vi "test json performance.vi"(8 "error in (no error)":errorcluster) -> (0 "error out":errorcluster, 1 "ms Avg Dump":dbl, 2 "ms Avg Load":dbl, 3 "Passed?":bool)   [LabVIEW 2019, in "labview_json_tests.lvlib"]
uses:
  labview_json_tests.lvlib
  lib/labview_json.lvlib
panel:
  out "Variant out":variant
  out "JSON out":string
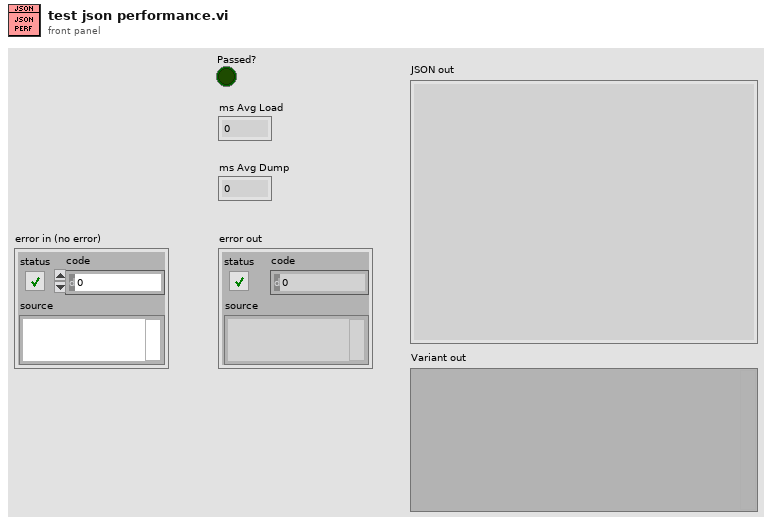
[diagram p1: front panel]
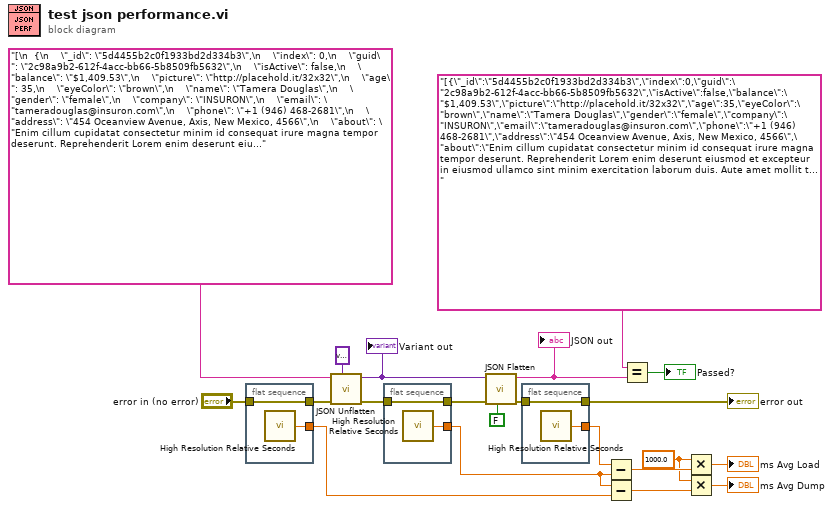
[diagram p0: block diagram]
diagram:
  w8 = 1000.0 ("x")
  n1 = flat-sequence {
    tunnel: [w23] -> w18
    tunnel: "error in (no error)" -> [w23]
    tunnel: [w22] -> w13
    frame #0 {
      n2 = call <vilib>:"High Resolution Relative Seconds.vi"() -> ("relative seconds"=w22:dbl)
    }
  }
  n3 = call "JSON Unflatten.vi"("Variant Type"=variant, "error in (no error)"=w18, "JSON in"="[\n  {\n    \"_id\": \"5d4455b2c0f1933bd2d334b3\",\n    \"index\": 0,\n    \"guid\": \"2c98a9b2-612f-4acc-bb66-5b8509fb5632\",\n    \"isActive\": false,\n    \"balance\": \"$1,409.53\",\n    \"picture\": \"http://placehold.it/32x32\",\n    \"age\": 35,\n    \"eyeColor\": \"brown\",\n    \"name\": \"Tamera Douglas\",\n    \"gender\": \"female\",\n    \"company\": \"INSURON\",\n    \"email\": \"tameradouglas@insuron.com\",\n    \"phone\": \"+1 (946) 468-2681\",\n    \"address\": \"454 Oceanview Avenue, Axis, New Mexico, 4566\",\n    \"about\": \"Enim cillum cupidatat consectetur minim id consequat irure magna tempor deserunt. Reprehenderit Lorem enim deserunt eiusmod et excepteur in eiusmod ullamco sint minim exercitation laborum duis. Aute amet mollit tempor adipisicing. Eiusmod tempor qui proident amet sint eiusmod laborum nisi consectetur. Excepteur occaecat et consequat pariatur pariatur sit deserunt proident commodo enim sit do. Duis fugiat irure esse ipsum non nulla ut aliquip esse nisi. Mollit commodo sit elit amet duis nisi sint.\",\n    \"registered\": \"2019-04-15T12:36:48 +06:00\",\n    \"latitude\": 7.38495,\n    \"longitude\": -44.890348,\n    \"tags\": [\n      \"cillum\",\n      \"nisi\",\n      \"mollit\",\n      \"sunt\",\n      \"minim\",\n      \"non\",\n      \"ex\"\n    ],\n    \"friends\": [\n      {\n        \"id\": 0,\n        \"name\": \"Winnie Reid\"\n      },\n      {\n        \"id\": 1,\n        \"name\": \"Araceli Delacruz\"\n      },\n      {\n        \"id\": 2,\n        \"name\": \"Bolton Horne\"\n      }\n    ],\n    \"greeting\": \"Hello, Tamera Douglas! You have 1 unread messages.\",\n    \"favoriteFruit\": \"banana\"\n  },\n  {\n    \"_id\": \"5d4455b247ae2b298863909d\",\n    \"index\": 1,\n    \"guid\": \"00a03766-a5ca-45cc-8dfb-1ef19cade6a5\",\n    \"isActive\": true,\n    \"balance\": \"$2,933.39\",\n    \"picture\": \"http://placehold.it/32x32\",\n    \"age\": 30,\n    \"eyeColor\": \"blue\",\n    \"name\": \"Garner Hooper\",\n    \"gender\": \"male\",\n    \"company\": \"SENMEI\",\n    \"email\": \"garnerhooper@senmei.com\",\n    \"phone\": \"+1 (805) 444-2443\",\n    \"address\": \"334 Herkimer Place, Westphalia, West Virginia, 8777\",\n    \"about\": \"Tempor tempor commodo do cillum ex. Velit minim esse nulla incididunt cupidatat. Aliqua tempor magna pariatur incididunt nostrud id cupidatat aliquip elit est ullamco. Mollit magna ut deserunt nisi exercitation reprehenderit proident ipsum occaecat ut enim. Voluptate adipisicing culpa veniam duis amet.\",\n    \"registered\": \"2019-02-20T09:03:35 +07:00\",\n    \"latitude\": 3.634789,\n    \"longitude\": -71.711449,\n    \"tags\": [\n      \"laboris\",\n      \"sunt\",\n      \"elit\",\n      \"esse\",\n      \"aliqua\",\n      \"nulla\",\n      \"in\"\n    ],\n    \"friends\": [\n      {\n        \"id\": 0,\n        \"name\": \"Saundra Mullen\"\n      },\n      {\n        \"id\": 1,\n        \"name\": \"Macdonald Houston\"\n      },\n      {\n        \"id\": 2,\n        \"name\": \"Rivera Hyde\"\n      }\n    ],\n    \"greeting\": \"Hello, Garner Hooper! You have 1 unread messages.\",\n    \"favoriteFruit\": \"banana\"\n  },\n  {\n    \"_id\": \"5d4455b288b3a8bcda8c1081\",\n    \"index\": 2,\n    \"guid\": \"14e7d77e-1ed5-4b08-bdae-19e0328d29f8\",\n    \"isActive\": false,\n    \"balance\": \"$1,321.03\",\n    \"picture\": \"http://placehold.it/32x32\",\n    \"age\": 33,\n    \"eyeColor\": \"blue\",\n    \"name\": \"Neal Buckley\",\n    \"gender\": \"male\",\n    \"company\": \"TRIBALOG\",\n    \"email\": \"nealbuckley@tribalog.com\",\n    \"phone\": \"+1 (879) 521-3254\",\n    \"address\": \"378 Preston Court, Unionville, Northern Mariana Islands, 6583\",\n    \"about\": \"Elit enim consectetur ad non tempor ad tempor proident do. In consectetur fugiat commodo ex. Ut nulla voluptate aliquip esse. Officia esse proident minim enim cillum deserunt mollit. Anim do deserunt amet velit consequat anim ullamco enim Lorem esse culpa irure voluptate labore. Laboris officia officia aliqua elit elit non culpa cillum dolore amet quis.\",\n    \"registered\": \"2019-01-23T03:40:45 +07:00\",\n    \"latitude\": 8.381404,\n    \"longitude\": -96.636286,\n    \"tags\": [\n      \"velit\",\n      \"esse\",\n      \"id\",\n      \"ullamco\",\n      \"sunt\",\n      \"amet\",\n      \"ad\"\n    ],\n    \"friends\": [\n      {\n        \"id\": 0,\n        \"name\": \"Hall Booker\"\n      },\n      {\n        \"id\": 1,\n        \"name\": \"Lawson Stevenson\"\n      },\n      {\n        \"id\": 2,\n        \"name\": \"Maynard Gill\"\n      }\n    ],\n    \"greeting\": \"Hello, Neal Buckley! You have 9 unread messages.\",\n    \"favoriteFruit\": \"apple\"\n  },\n  {\n    \"_id\": \"5d4455b21a3db63bef3f777a\",\n    \"index\": 3,\n    \"guid\": \"d4ea16a6-f1ec-4bfe-9970-657798a14ac1\",\n    \"isActive\": false,\n    \"balance\": \"$2,499.94\",\n    \"picture\": \"http://placehold.it/32x32\",\n    \"age\": 37,\n    \"eyeColor\": \"green\",\n    \"name\": \"Marguerite Gay\",\n    \"gender\": \"female\",\n    \"company\": \"DADABASE\",\n    \"email\": \"margueritegay@dadabase.com\",\n    \"phone\": \"+1 (937) 434-3754\",\n    \"address\": \"256 Dooley Street, Sylvanite, Nevada, 1343\",\n    \"about\": \"Aute elit laborum cillum minim esse ex eu est. Cillum in esse irure ut do duis et eiusmod aliqua et adipisicing. Sunt adipisicing commodo dolor sit qui laborum commodo deserunt amet minim. Proident sint labore consequat commodo enim veniam veniam ea amet eu qui. Officia culpa dolor adipisicing laborum. Commodo elit sunt anim laboris laborum amet nulla.\",\n    \"registered\": \"2014-05-27T12:57:25 +06:00\",\n    \"latitude\": 64.083884,\n    \"longitude\": -30.078651,\n    \"tags\": [\n      \"minim\",\n      \"mollit\",\n      \"laboris\",\n      \"pariatur\",\n      \"qui\",\n      \"sit\",\n      \"do\"\n    ],\n    \"friends\": [\n      {\n        \"id\": 0,\n        \"name\": \"Duffy Steele\"\n      },\n      {\n        \"id\": 1,\n        \"name\": \"Preston Lamb\"\n      },\n      {\n        \"id\": 2,\n        \"name\": \"Velasquez Shaffer\"\n      }\n    ],\n    \"greeting\": \"Hello, Marguerite Gay! You have 5 unread messages.\",\n    \"favoriteFruit\": \"apple\"\n  },\n  {\n    \"_id\": \"5d4455b2664446faf7994a00\",\n    \"index\": 4,\n    \"guid\": \"75fe4cd8-2ec4-47e4-9a35-4a72f803cd01\",\n    \"isActive\": true,\n    \"balance\": \"$3,522.35\",\n    \"picture\": \"http://placehold.it/32x32\",\n    \"age\": 20,\n    \"eyeColor\": \"brown\",\n    \"name\": \"Graciela Orr\",\n    \"gender\": \"female\",\n    \"company\": \"ENTROFLEX\",\n    \"email\": \"gracielaorr@entroflex.com\",\n    \"phone\": \"+1 (855) 541-3462\",\n    \"address\": \"895 Sapphire Street, Ruckersville, Georgia, 6484\",\n    \"about\": \"Consectetur reprehenderit laboris minim anim aute aliquip Lorem ullamco non consequat. Tempor officia occaecat eu amet quis quis fugiat. Eu ad ex elit dolor. Do proident veniam aute irure consectetur laborum nulla qui Lorem ut culpa commodo. Quis commodo commodo sint sunt veniam. Magna commodo reprehenderit duis eu deserunt qui amet. Pariatur ut occaecat minim officia commodo voluptate esse in id anim.\",\n    \"registered\": \"2017-02-22T08:24:12 +07:00\",\n    \"latitude\": -84.018578,\n    \"longitude\": 66.386099,\n    \"tags\": [\n      \"excepteur\",\n      \"anim\",\n      \"commodo\",\n      \"amet\",\n      \"consequat\",\n      \"tempor\",\n      \"quis\"\n    ],\n    \"friends\": [\n      {\n        \"id\": 0,\n        \"name\": \"Ollie Cline\"\n      },\n      {\n        \"id\": 1,\n        \"name\": \"Corina Powers\"\n      },\n      {\n        \"id\": 2,\n        \"name\": \"Lynda Workman\"\n      }\n    ],\n    \"greeting\": \"Hello, Graciela Orr! You have 6 unread messages.\",\n    \"favoriteFruit\": \"apple\"\n  },\n  {\n    \"_id\": \"5d4455b2ca59b0a7fc9c71cd\",\n    \"index\": 5,\n    \"guid\": \"a5d705b7-9c22-4a73-968c-37b6847d31de\",\n    \"isActive\": true,\n    \"balance\": \"$2,719.98\",\n    \"picture\": \"http://placehold.it/32x32\",\n    \"age\": 30,\n    \"eyeColor\": \"blue\",\n    \"name\": \"Lynn Durham\",\n    \"gender\": \"male\",\n    \"company\": \"RODEOMAD\",\n    \"email\": \"lynndurham@rodeomad.com\",\n    \"phone\": \"+1 (896) 522-2325\",\n    \"address\": \"202 Erskine Loop, Silkworth, North Dakota, 8325\",\n    \"about\": \"Anim sunt irure ut sint. Ullamco consectetur non pariatur consectetur ullamco. Consequat cupidatat nisi eiusmod magna ut eiusmod. Ullamco cillum culpa voluptate fugiat laboris nulla Lorem ad irure ipsum mollit.\",\n    \"registered\": \"2017-06-19T08:42:14 +06:00\",\n    \"latitude\": -19.936145,\n    \"longitude\": 149.259571,\n    \"tags\": [\n      \"ea\",\n      \"proident\",\n      \"tempor\",\n      \"cillum\",\n      \"sit\",\n      \"veniam\",\n      \"velit\"\n    ],\n    \"friends\": [\n      {\n        \"id\": 0,\n        \"name\": \"Horne Kelley\"\n      },\n      {\n        \"id\": 1,\n        \"name\": \"Elvia Harper\"\n      },\n      {\n        \"id\": 2,\n        \"name\": \"Hooper Griffith\"\n      }\n    ],\n    \"greeting\": \"Hello, Lynn Durham! You have 2 unread messages.\",\n    \"favoriteFruit\": \"banana\"\n  },\n  {\n    \"_id\": \"5d4455b2293b6080ad5e354a\",\n    \"index\": 6,\n    \"guid\": \"64e7c98c-aecf-4ff2-aeff-e95c9629e4fa\",\n    \"isActive\": false,\n    \"balance\": \"$3,702.37\",\n    \"picture\": \"http://placehold.it/32x32\",\n    \"age\": 22,\n    \"eyeColor\": \"brown\",\n    \"name\": \"Bethany Salazar\",\n    \"gender\": \"female\",\n    \"company\": \"TRIPSCH\",\n    \"email\": \"bethanysalazar@tripsch.com\",\n    \"phone\": \"+1 (856) 524-3649\",\n    \"address\": \"754 Prospect Place, Crumpler, Palau, 1899\",\n    \"about\": \"Tempor non occaecat veniam non. Mollit exercitation magna eiusmod cillum. Consequat do irure deserunt velit. Consectetur aute deserunt esse anim nostrud do.\",\n    \"registered\": \"2014-09-10T09:21:42 +06:00\",\n    \"latitude\": -55.3388,\n    \"longitude\": -63.497523,\n    \"tags\": [\n      \"incididunt\",\n      \"cupidatat\",\n      \"voluptate\",\n      \"pariatur\",\n      \"dolore\",\n      \"tempor\",\n      \"laborum\"\n    ],\n    \"friends\": [\n      {\n        \"id\": 0,\n        \"name\": \"Weiss Hahn\"\n      },\n      {\n        \"id\": 1,\n        \"name\": \"Trudy Roy\"\n      },\n      {\n        \"id\": 2,\n        \"name\": \"Schultz Vazquez\"\n      }\n    ],\n    \"greeting\": \"Hello, Bethany Salazar! You have 4 unread messages.\",\n    \"favoriteFruit\": \"banana\"\n  }\n]" ("JSON")) -> ("error out"=w17:errorcluster, "Variant out"=w14:variant)  [unwired: 6 in, 1 out]
  "Variant out" <- w14
  n4 = flat-sequence {
    tunnel: [w25] -> w16
    tunnel: w17 -> [w25]
    tunnel: [w24] -> w11
    frame #0 {
      n5 = call <vilib>:"High Resolution Relative Seconds.vi"() -> ("relative seconds"=w24:dbl)
    }
  }
  n6 = call "JSON Flatten.vi"("Pretty Print? (F)"=FALSE, "error in (no error)"=w16, "Variant in"=w14) -> ("error out"=w15:errorcluster, "JSON out"=w20:string)  [unwired: 7 in]
  "JSON out" <- w20
  n7 = flat-sequence {
    tunnel: [w27] -> w2
    tunnel: w15 -> [w27]
    tunnel: [w26] -> w12
    frame #0 {
      n8 = call <vilib>:"High Resolution Relative Seconds.vi"() -> ("relative seconds"=w26:dbl)
    }
  }
  n9 = Subtract(x=w12, y=w11) -> (x-y=w10:dbl)
  n10 = Subtract(x=w11, y=w13) -> (x-y=w9:dbl)
  n11 = Equal?(x="[{\"_id\":\"5d4455b2c0f1933bd2d334b3\",\"index\":0,\"guid\":\"2c98a9b2-612f-4acc-bb66-5b8509fb5632\",\"isActive\":false,\"balance\":\"$1,409.53\",\"picture\":\"http://placehold.it/32x32\",\"age\":35,\"eyeColor\":\"brown\",\"name\":\"Tamera Douglas\",\"gender\":\"female\",\"company\":\"INSURON\",\"email\":\"tameradouglas@insuron.com\",\"phone\":\"+1 (946) 468-2681\",\"address\":\"454 Oceanview Avenue, Axis, New Mexico, 4566\",\"about\":\"Enim cillum cupidatat consectetur minim id consequat irure magna tempor deserunt. Reprehenderit Lorem enim deserunt eiusmod et excepteur in eiusmod ullamco sint minim exercitation laborum duis. Aute amet mollit tempor adipisicing. Eiusmod tempor qui proident amet sint eiusmod laborum nisi consectetur. Excepteur occaecat et consequat pariatur pariatur sit deserunt proident commodo enim sit do. Duis fugiat irure esse ipsum non nulla ut aliquip esse nisi. Mollit commodo sit elit amet duis nisi sint.\",\"registered\":\"2019-04-15T12:36:48 +06:00\",\"latitude\":7.38495,\"longitude\":-44.890348,\"tags\":[\"cillum\",\"nisi\",\"mollit\",\"sunt\",\"minim\",\"non\",\"ex\"],\"friends\":[{\"id\":0,\"name\":\"Winnie Reid\"},{\"id\":1,\"name\":\"Araceli Delacruz\"},{\"id\":2,\"name\":\"Bolton Horne\"}],\"greeting\":\"Hello, Tamera Douglas! You have 1 unread messages.\",\"favoriteFruit\":\"banana\"},{\"_id\":\"5d4455b247ae2b298863909d\",\"index\":1,\"guid\":\"00a03766-a5ca-45cc-8dfb-1ef19cade6a5\",\"isActive\":true,\"balance\":\"$2,933.39\",\"picture\":\"http://placehold.it/32x32\",\"age\":30,\"eyeColor\":\"blue\",\"name\":\"Garner Hooper\",\"gender\":\"male\",\"company\":\"SENMEI\",\"email\":\"garnerhooper@senmei.com\",\"phone\":\"+1 (805) 444-2443\",\"address\":\"334 Herkimer Place, Westphalia, West Virginia, 8777\",\"about\":\"Tempor tempor commodo do cillum ex. Velit minim esse nulla incididunt cupidatat. Aliqua tempor magna pariatur incididunt nostrud id cupidatat aliquip elit est ullamco. Mollit magna ut deserunt nisi exercitation reprehenderit proident ipsum occaecat ut enim. Voluptate adipisicing culpa veniam duis amet.\",\"registered\":\"2019-02-20T09:03:35 +07:00\",\"latitude\":3.634789,\"longitude\":-71.711449,\"tags\":[\"laboris\",\"sunt\",\"elit\",\"esse\",\"aliqua\",\"nulla\",\"in\"],\"friends\":[{\"id\":0,\"name\":\"Saundra Mullen\"},{\"id\":1,\"name\":\"Macdonald Houston\"},{\"id\":2,\"name\":\"Rivera Hyde\"}],\"greeting\":\"Hello, Garner Hooper! You have 1 unread messages.\",\"favoriteFruit\":\"banana\"},{\"_id\":\"5d4455b288b3a8bcda8c1081\",\"index\":2,\"guid\":\"14e7d77e-1ed5-4b08-bdae-19e0328d29f8\",\"isActive\":false,\"balance\":\"$1,321.03\",\"picture\":\"http://placehold.it/32x32\",\"age\":33,\"eyeColor\":\"blue\",\"name\":\"Neal Buckley\",\"gender\":\"male\",\"company\":\"TRIBALOG\",\"email\":\"nealbuckley@tribalog.com\",\"phone\":\"+1 (879) 521-3254\",\"address\":\"378 Preston Court, Unionville, Northern Mariana Islands, 6583\",\"about\":\"Elit enim consectetur ad non tempor ad tempor proident do. In consectetur fugiat commodo ex. Ut nulla voluptate aliquip esse. Officia esse proident minim enim cillum deserunt mollit. Anim do deserunt amet velit consequat anim ullamco enim Lorem esse culpa irure voluptate labore. Laboris officia officia aliqua elit elit non culpa cillum dolore amet quis.\",\"registered\":\"2019-01-23T03:40:45 +07:00\",\"latitude\":8.381404,\"longitude\":-96.636286,\"tags\":[\"velit\",\"esse\",\"id\",\"ullamco\",\"sunt\",\"amet\",\"ad\"],\"friends\":[{\"id\":0,\"name\":\"Hall Booker\"},{\"id\":1,\"name\":\"Lawson Stevenson\"},{\"id\":2,\"name\":\"Maynard Gill\"}],\"greeting\":\"Hello, Neal Buckley! You have 9 unread messages.\",\"favoriteFruit\":\"apple\"},{\"_id\":\"5d4455b21a3db63bef3f777a\",\"index\":3,\"guid\":\"d4ea16a6-f1ec-4bfe-9970-657798a14ac1\",\"isActive\":false,\"balance\":\"$2,499.94\",\"picture\":\"http://placehold.it/32x32\",\"age\":37,\"eyeColor\":\"green\",\"name\":\"Marguerite Gay\",\"gender\":\"female\",\"company\":\"DADABASE\",\"email\":\"margueritegay@dadabase.com\",\"phone\":\"+1 (937) 434-3754\",\"address\":\"256 Dooley Street, Sylvanite, Nevada, 1343\",\"about\":\"Aute elit laborum cillum minim esse ex eu est. Cillum in esse irure ut do duis et eiusmod aliqua et adipisicing. Sunt adipisicing commodo dolor sit qui laborum commodo deserunt amet minim. Proident sint labore consequat commodo enim veniam veniam ea amet eu qui. Officia culpa dolor adipisicing laborum. Commodo elit sunt anim laboris laborum amet nulla.\",\"registered\":\"2014-05-27T12:57:25 +06:00\",\"latitude\":64.083884,\"longitude\":-30.078651,\"tags\":[\"minim\",\"mollit\",\"laboris\",\"pariatur\",\"qui\",\"sit\",\"do\"],\"friends\":[{\"id\":0,\"name\":\"Duffy Steele\"},{\"id\":1,\"name\":\"Preston Lamb\"},{\"id\":2,\"name\":\"Velasquez Shaffer\"}],\"greeting\":\"Hello, Marguerite Gay! You have 5 unread messages.\",\"favoriteFruit\":\"apple\"},{\"_id\":\"5d4455b2664446faf7994a00\",\"index\":4,\"guid\":\"75fe4cd8-2ec4-47e4-9a35-4a72f803cd01\",\"isActive\":true,\"balance\":\"$3,522.35\",\"picture\":\"http://placehold.it/32x32\",\"age\":20,\"eyeColor\":\"brown\",\"name\":\"Graciela Orr\",\"gender\":\"female\",\"company\":\"ENTROFLEX\",\"email\":\"gracielaorr@entroflex.com\",\"phone\":\"+1 (855) 541-3462\",\"address\":\"895 Sapphire Street, Ruckersville, Georgia, 6484\",\"about\":\"Consectetur reprehenderit laboris minim anim aute aliquip Lorem ullamco non consequat. Tempor officia occaecat eu amet quis quis fugiat. Eu ad ex elit dolor. Do proident veniam aute irure consectetur laborum nulla qui Lorem ut culpa commodo. Quis commodo commodo sint sunt veniam. Magna commodo reprehenderit duis eu deserunt qui amet. Pariatur ut occaecat minim officia commodo voluptate esse in id anim.\",\"registered\":\"2017-02-22T08:24:12 +07:00\",\"latitude\":-84.018578,\"longitude\":66.386099,\"tags\":[\"excepteur\",\"anim\",\"commodo\",\"amet\",\"consequat\",\"tempor\",\"quis\"],\"friends\":[{\"id\":0,\"name\":\"Ollie Cline\"},{\"id\":1,\"name\":\"Corina Powers\"},{\"id\":2,\"name\":\"Lynda Workman\"}],\"greeting\":\"Hello, Graciela Orr! You have 6 unread messages.\",\"favoriteFruit\":\"apple\"},{\"_id\":\"5d4455b2ca59b0a7fc9c71cd\",\"index\":5,\"guid\":\"a5d705b7-9c22-4a73-968c-37b6847d31de\",\"isActive\":true,\"balance\":\"$2,719.98\",\"picture\":\"http://placehold.it/32x32\",\"age\":30,\"eyeColor\":\"blue\",\"name\":\"Lynn Durham\",\"gender\":\"male\",\"company\":\"RODEOMAD\",\"email\":\"lynndurham@rodeomad.com\",\"phone\":\"+1 (896) 522-2325\",\"address\":\"202 Erskine Loop, Silkworth, North Dakota, 8325\",\"about\":\"Anim sunt irure ut sint. Ullamco consectetur non pariatur consectetur ullamco. Consequat cupidatat nisi eiusmod magna ut eiusmod. Ullamco cillum culpa voluptate fugiat laboris nulla Lorem ad irure ipsum mollit.\",\"registered\":\"2017-06-19T08:42:14 +06:00\",\"latitude\":-19.936145,\"longitude\":149.259571,\"tags\":[\"ea\",\"proident\",\"tempor\",\"cillum\",\"sit\",\"veniam\",\"velit\"],\"friends\":[{\"id\":0,\"name\":\"Horne Kelley\"},{\"id\":1,\"name\":\"Elvia Harper\"},{\"id\":2,\"name\":\"Hooper Griffith\"}],\"greeting\":\"Hello, Lynn Durham! You have 2 unread messages.\",\"favoriteFruit\":\"banana\"},{\"_id\":\"5d4455b2293b6080ad5e354a\",\"index\":6,\"guid\":\"64e7c98c-aecf-4ff2-aeff-e95c9629e4fa\",\"isActive\":false,\"balance\":\"$3,702.37\",\"picture\":\"http://placehold.it/32x32\",\"age\":22,\"eyeColor\":\"brown\",\"name\":\"Bethany Salazar\",\"gender\":\"female\",\"company\":\"TRIPSCH\",\"email\":\"bethanysalazar@tripsch.com\",\"phone\":\"+1 (856) 524-3649\",\"address\":\"754 Prospect Place, Crumpler, Palau, 1899\",\"about\":\"Tempor non occaecat veniam non. Mollit exercitation magna eiusmod cillum. Consequat do irure deserunt velit. Consectetur aute deserunt esse anim nostrud do.\",\"registered\":\"2014-09-10T09:21:42 +06:00\",\"latitude\":-55.3388,\"longitude\":-63.497523,\"tags\":[\"incididunt\",\"cupidatat\",\"voluptate\",\"pariatur\",\"dolore\",\"tempor\",\"laborum\"],\"friends\":[{\"id\":0,\"name\":\"Weiss Hahn\"},{\"id\":1,\"name\":\"Trudy Roy\"},{\"id\":2,\"name\":\"Schultz Vazquez\"}],\"greeting\":\"Hello, Bethany Salazar! You have 4 unread messages.\",\"favoriteFruit\":\"banana\"}]" ("JSON"), y=w20) -> (x = y?=→"Passed?":bool)
  n12 = Multiply(x=w8, y=w10) -> (x*y=→"ms Avg Load":dbl)
  n13 = Multiply(x=w8, y=w9) -> (x*y=→"ms Avg Dump":dbl)
  "error out" <- w2
